vi "setUp.vi"(8 "error in (no error)":errorcluster, 11 "reference in":refnum<class "Configure Filter Unit Test.lvclass">) -> (0 "error out":errorcluster, 3 "reference out":refnum<class "Configure Filter Unit Test.lvclass">)   [LabVIEW 2016, in "Configure Filter Unit Test.lvclass"]
doc: "setUp runs prior to the test method during test execution. Use this method to initialize any object data required by your tests."
uses:
  Configure Filter Unit Test.lvclass
  C:/Program Files (x86)/National Instruments/LabVIEW 2016/vi.lib/addons/_JKI Toolkits/VI Tester/TestCase.llb/TestCase.lvclass
  Configure Filter Unit Test.lvclass/Configure Filter Unit Test.ctl
  <vilib>/addons/_JKI Toolkits/VI Tester/TestCase.llb/TestCase.lvclass
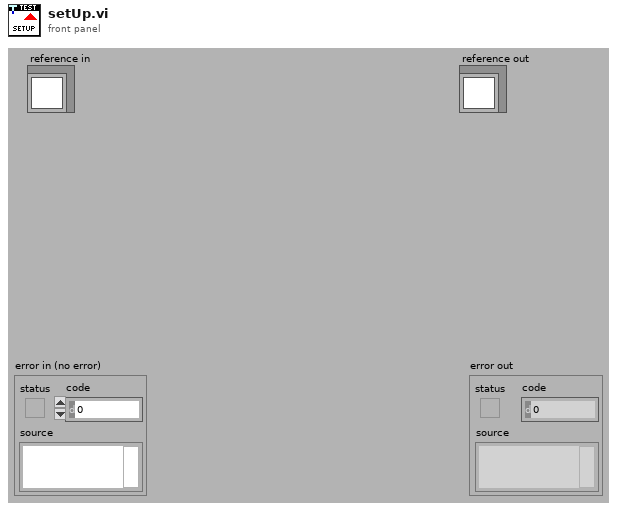
[diagram p1: front panel]
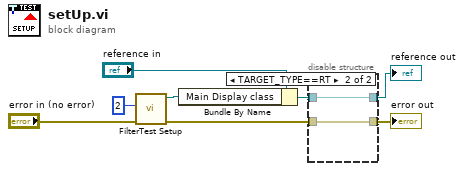
[diagram p0: block diagram]
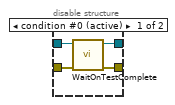
[diagram p2: hidden frame]
diagram:
  n1 = call "FilterTest Setup.vi"("error in (no error)"="error in (no error)", "Number of Test Filters"=2) -> ("error out"=w1:errorcluster, "Main Display out"=w3:refnum<class "Main Display.lvclass">)  [unwired: 8 in]
  n2 = Bundle By Name(cluster="reference in", "Main Display class"=w3) -> (w5:refnum<class "Configure Filter Unit Test.lvclass">)
  n3 = disable-structure shown="TARGET_TYPE==RT" {
    disable-tunnel: w1 -> [w12 w13]
    disable-tunnel: [w11 w13] -> w8
    disable-tunnel: [w10 w14] -> w6
    disable-tunnel: w5 -> [w9 w14]
    frame condition #0 (active) {
      n4 = call <vilib>:"WaitOnTestComplete.vi"("error in (no error)"=w12, "TestCase in"=w9) -> ("error out"=w11:errorcluster, "TestCase out"=w10:refnum<class "Configure Filter Unit Test.lvclass">)  [unwired: 8 in]
    }
    frame condition #1 {
    }
  }
  "error out" <- w8
  "reference out" <- w6
